vi "002_NBT Testplatform V3.1.vi"(11 "Queue Ref In":T1={"UI"=refnum, "Message"=refnum, "Data"=refnum, "Caller"=refnum, "Name"="000 Common", "Data Path"=path "", "Class Path"=path "", "SubPanel"=refnum, "Project Name"="", "MNT"="", "Title"="", "Data Source"=refnum, "Queue List"={}, "VI"=refnum, "UE"=refnum}) -> ()   [LabVIEW 2020]
doc: "000001"
uses:
  Alin/QMH/000 Module Data Type.ctl
  Alin/QMH/Queue Message.ctl
  <vilib>/Utility/file.llb/Read Delimited Spreadsheet (string).vi
  <vilib>/Utility/file.llb/Write Delimited Spreadsheet (string).vi
  <vilib>/Utility/cursorutil.llb/Set Cursor (Icon Pict).vi
  <vilib>/Utility/config.llb/Read Key (String).vi
  <vilib>/Utility/config.llb/NI_LVConfig.lvlib
panel:
  in  "Data Source Manage":bool
  out "Logo":picture
  out "Title":string="AlinFramwork Test"
  out "Warning":bool
  in  "User":string="你好！管理员 Debug"
  out "Log":string
  in  "Warning Record":string
  out "字符串":string
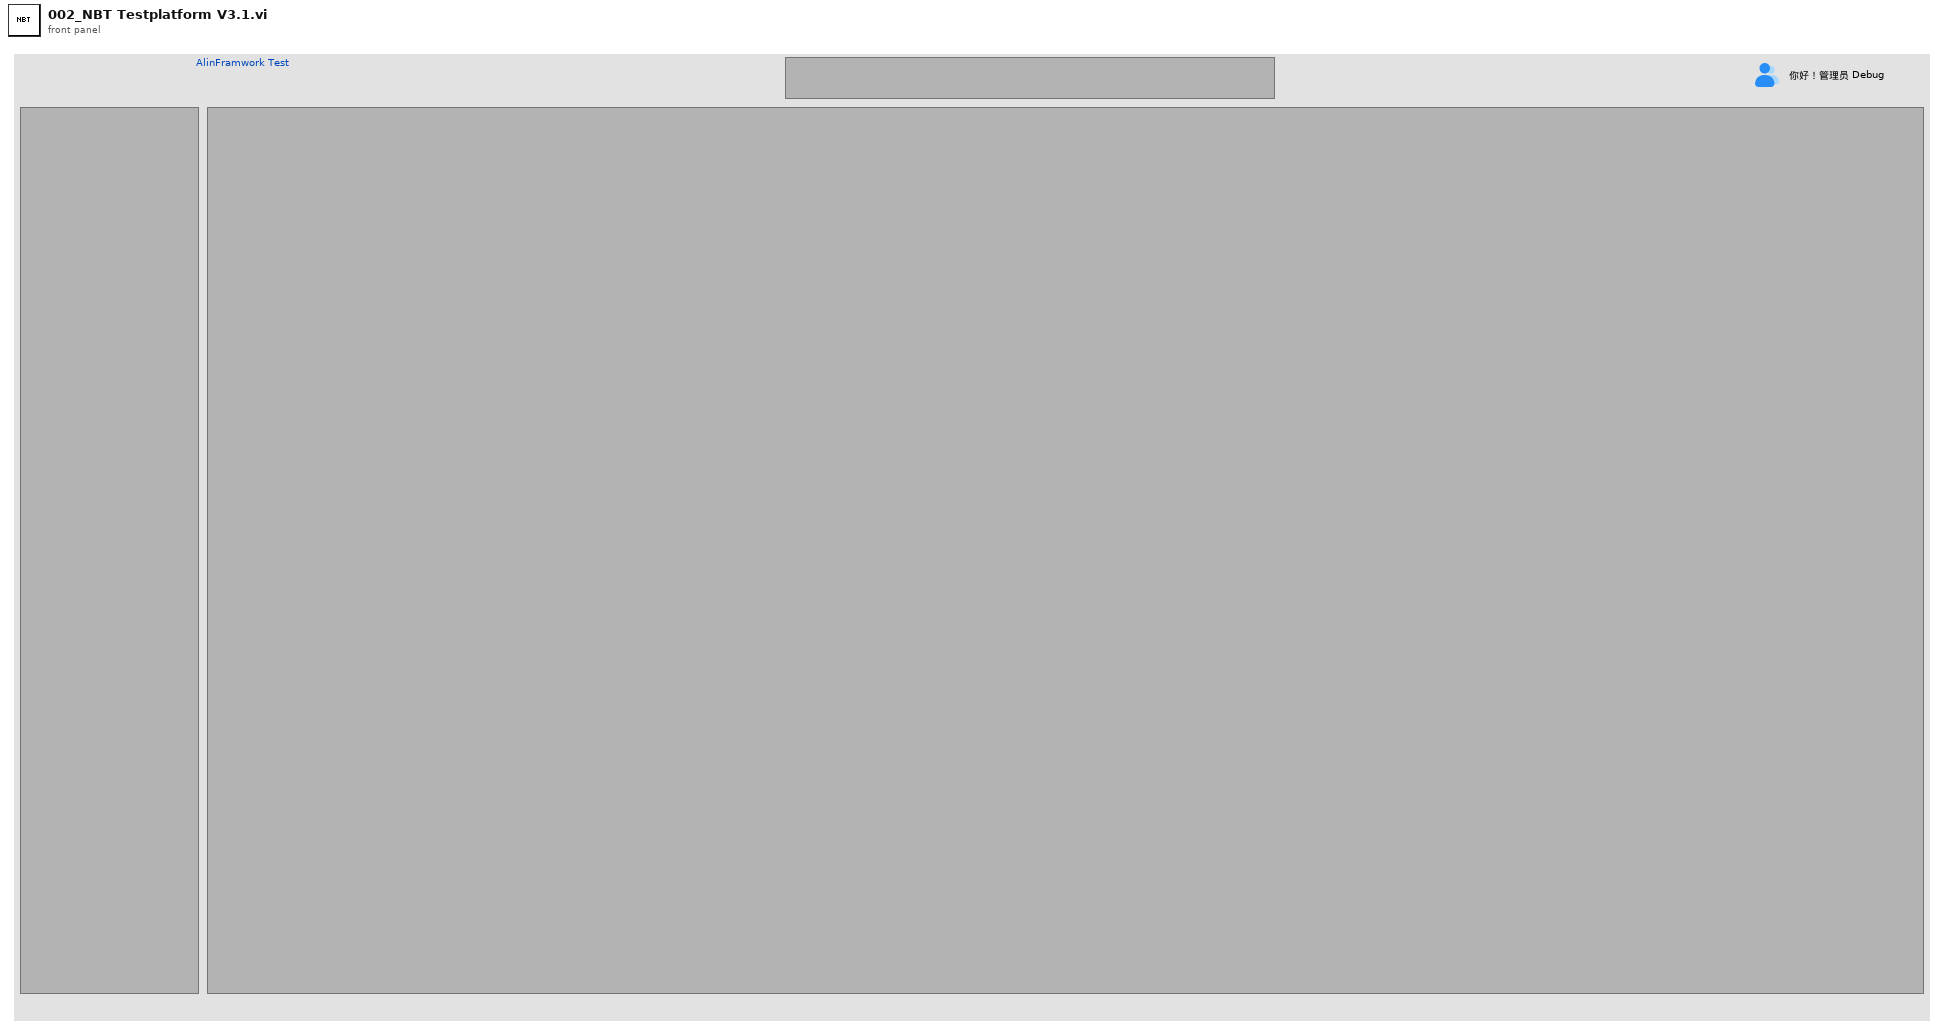
[diagram p1: front panel]
types:
  T1 = typedef "000 Module Data Type.ctl" = cluster{"UI":refnum<queue>, "Message":refnum<queue>, "Data":refnum<queue>, "Caller":refnum<queue>, "Name":string, "Data Path":path, "Class Path":path, "SubPanel":refnum<vi>, "Project Name":string, "MNT":string, "Title":string, "Data Source":refnum<queue>, "Queue List":map{string, refnum<queue>}, "VI":refnum<vi>, "UE":refnum<user-event>}
  T2 = cluster{"Interval":cluster{"min":i32, "max":i32}, "Color":cluster{"off":u32, "on":u32}, "Panel":cluster{"Panel01":bool, "Panel02":bool, "Panel03":bool, "Panel04":bool, "Panel05":bool, "Panel06":bool, "Panel07":bool}, "SubPanel":cluster{"Panel01":refnum<vi>, "Panel02":refnum<vi>, "Panel03":refnum<vi>, "Panel04":refnum<vi>, "Panel05":refnum<vi>, "Panel06":refnum<vi>, "Panel07":refnum<vi>}, "Queue Ref ":T1, "Panel Name":string[], "Write":map{string, string}, "Warning":refnum<vi>, "Info":cluster{"Title":string, "Names":string[], "Logo":string}, "Panel Config":bool, "Spliter":refnum<vi>, "Log Name":string, "Last":i32}
  T3 = typedef "NI_LVConfig.lvlib/Config Data RefNum.ctl" = refnum<k1>
  T4 = typedef "imagedata.ctl" = cluster{"image type":i32, "image depth":i32, "image":u8[], "mask":u8[], "colors":u32[], "Rectangle":cluster{"left":i16, "top":i16, "right":i16, "bottom":i16}}
  T5 = cluster{"Panel01":refnum<vi>, "Panel02":refnum<vi>, "Panel03":refnum<vi>, "Panel04":refnum<vi>, "Panel05":refnum<vi>, "Panel06":refnum<vi>, "Panel07":refnum<vi>}
  T6 = enum32{"invalid app kind", "Development System", "Run Time System", "Student Edition", "Embedded LabVIEW", "Evaluation", "Custom"}
  T7 = typedef "eventvkey.ctl" = enum16{"ASCII", "Enter", "Return", "Shift", "Ctrl", "Alt", "Cmd", "Opt", "Caps", "NumLock", "Clear", "Break", "Up", "Down", "Left", "Right", "Insert", "Delete", "Home", "End", "PageUp", "PageDown", "Escape", "Help", "Pause", "ScrollLock", "F1", "F2", "F3", "F4", "F5", "F6", "F7", "F8", "F9", "F10", "F11", "F12", "F13", "F14", "F15", "F16", "F17", "F18", "F19", "F20", "F21", "F22", "F23", "F24", "Play", "VolumeUp", "VolumeDown", "Mute", "Two Byte Char"}
  T8 = cluster{"Shift":bool, "Ctrl":bool, "Alt":bool, "Cmd":bool, "Opt":bool}
  T9 = cluster{"Queue Ref":T1, "Queue List":map{string, refnum<queue>}, "Panel Adjust":string, "Panel Name":string[], "Panel Info":map{string, cluster{"Lable":string, "Name":string, "Panel":string, "Use":string}}, "SubPanel":refnum<vi>}
  T10 = map{string, cluster{"Lable":string, "Name":string, "Panel":string, "Use":string}}
  T11 = cluster{"Lable":string, "Name":string, "Panel":string, "Use":string}
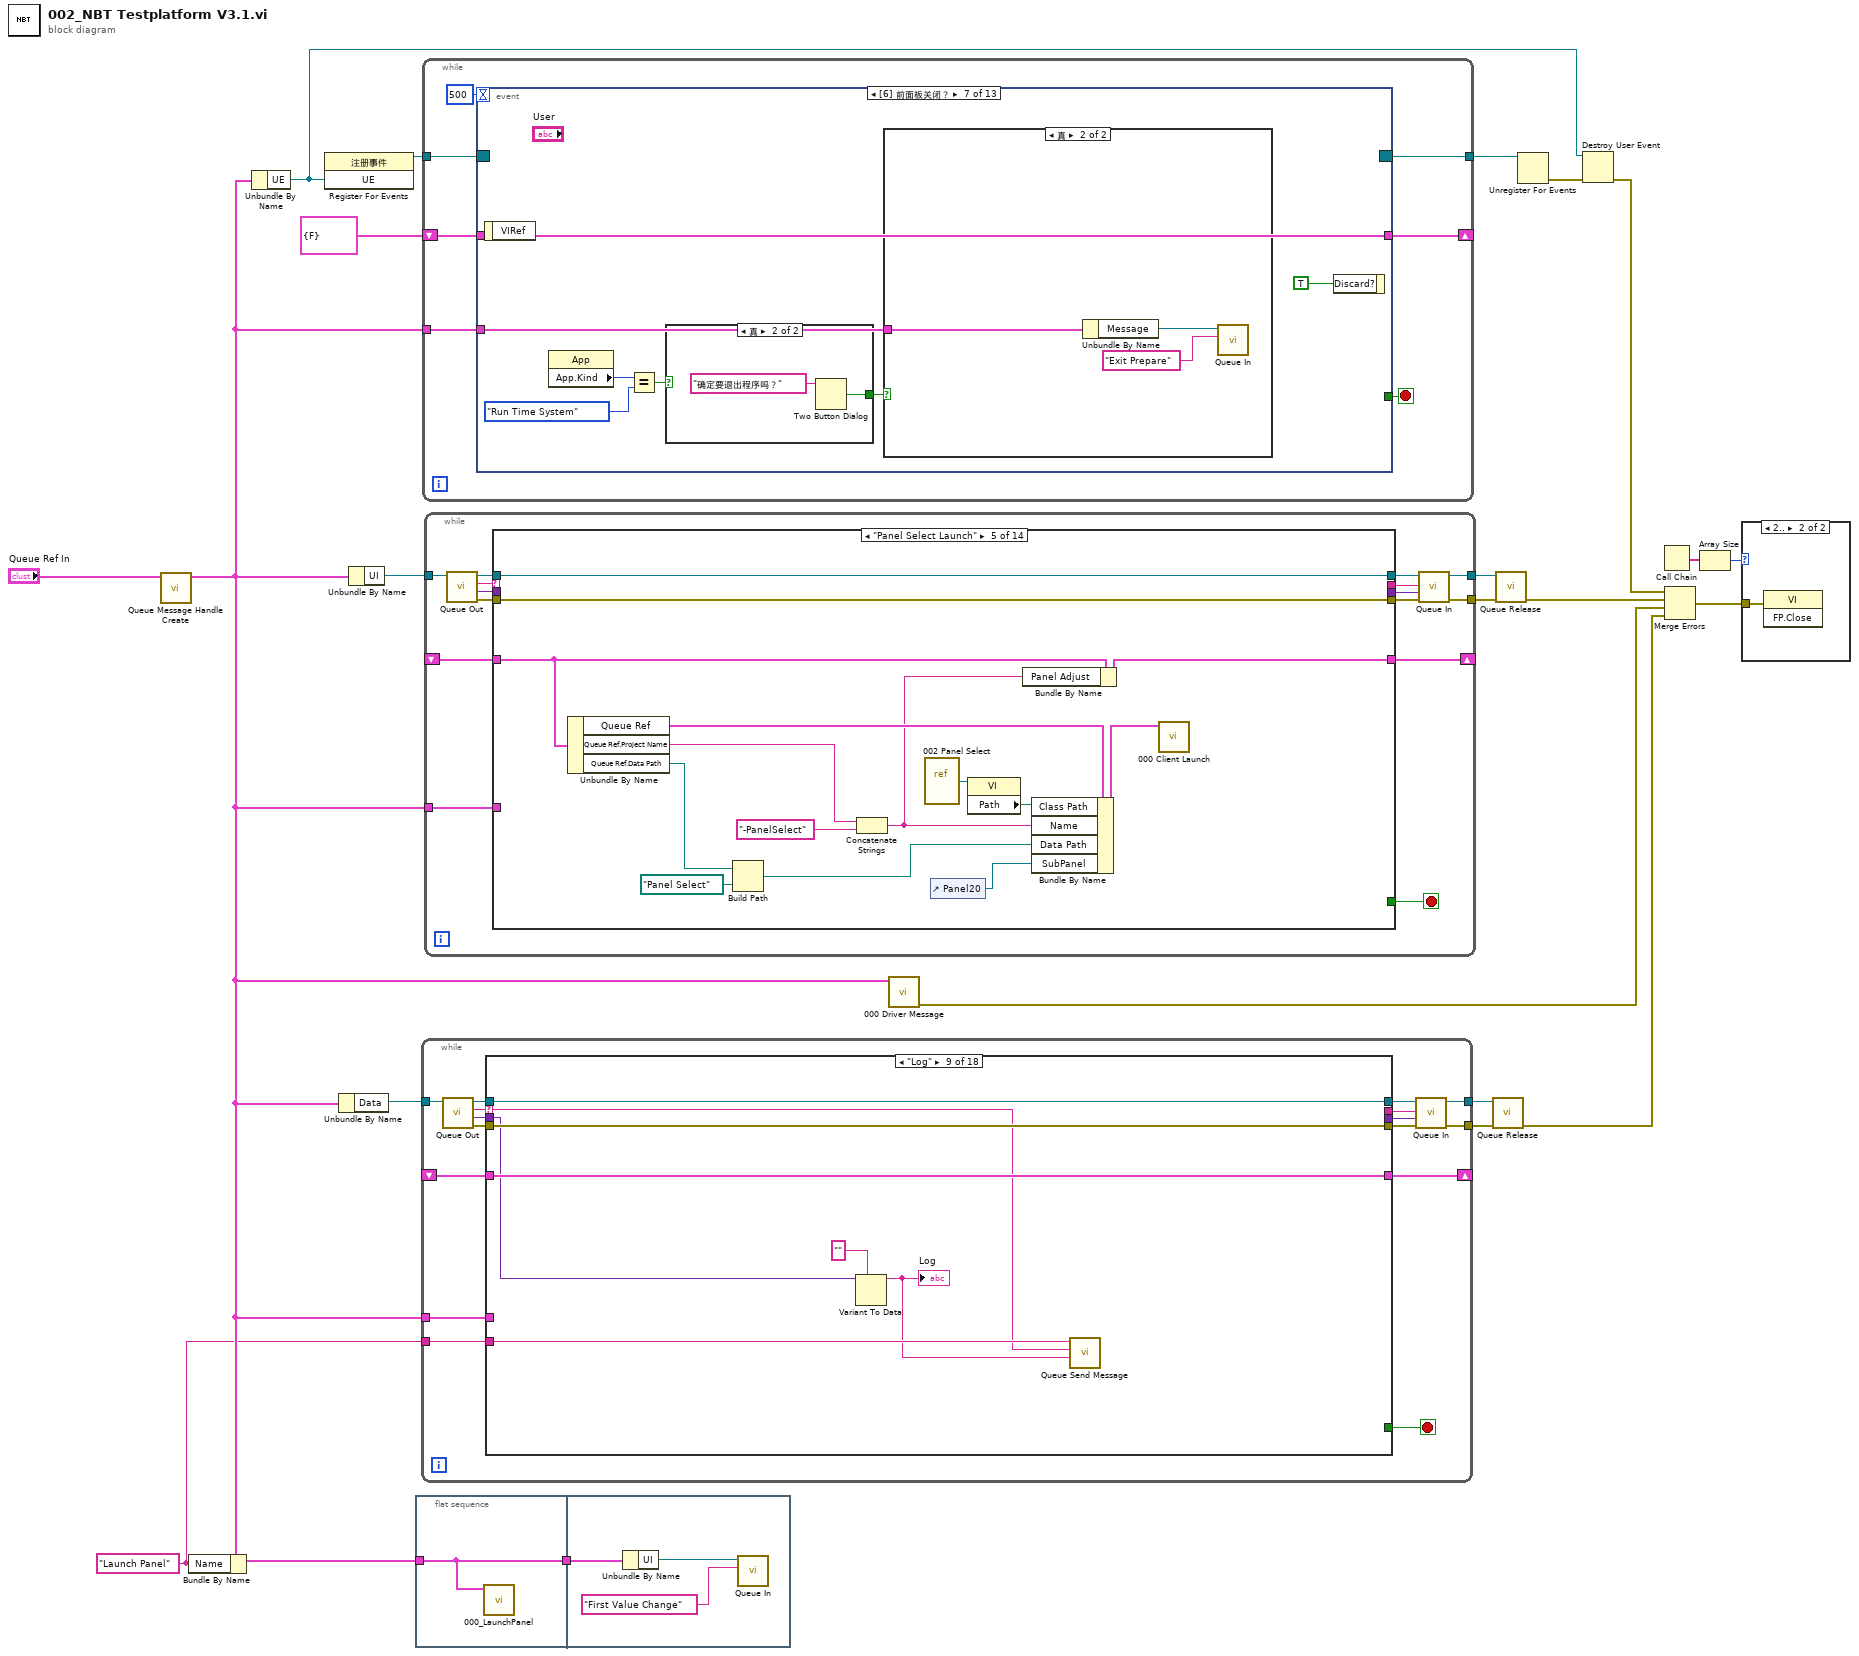
[diagram p0: block diagram]
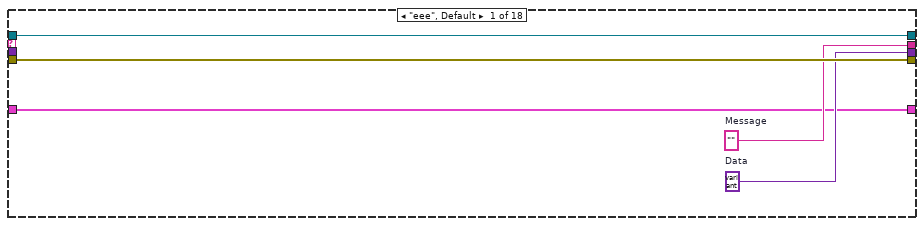
[diagram p2: hidden frame]
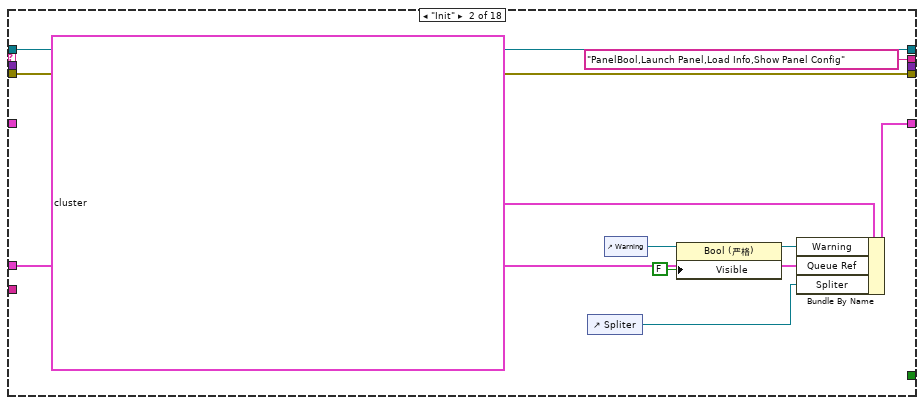
[diagram p3: hidden frame]
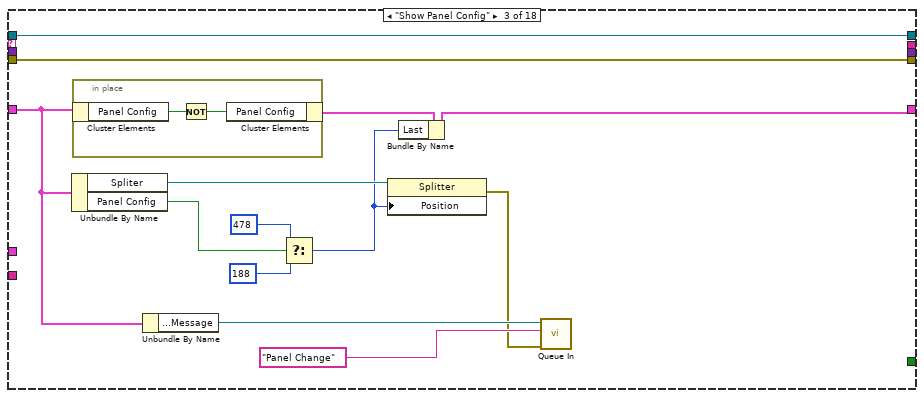
[diagram p4: hidden frame]
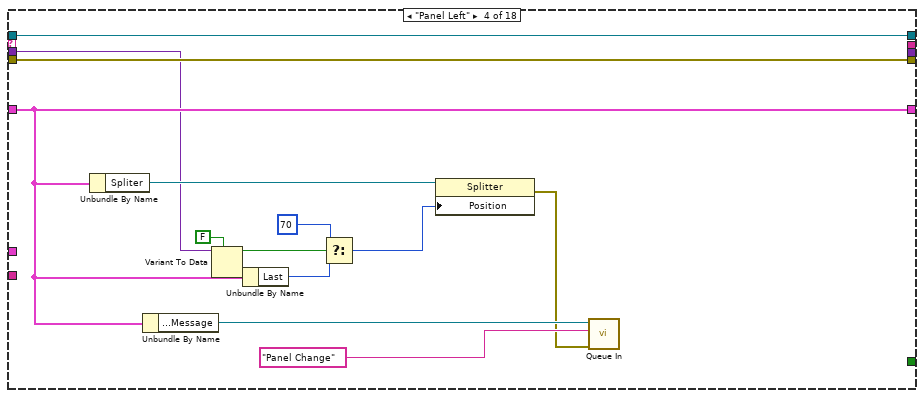
[diagram p5: hidden frame]
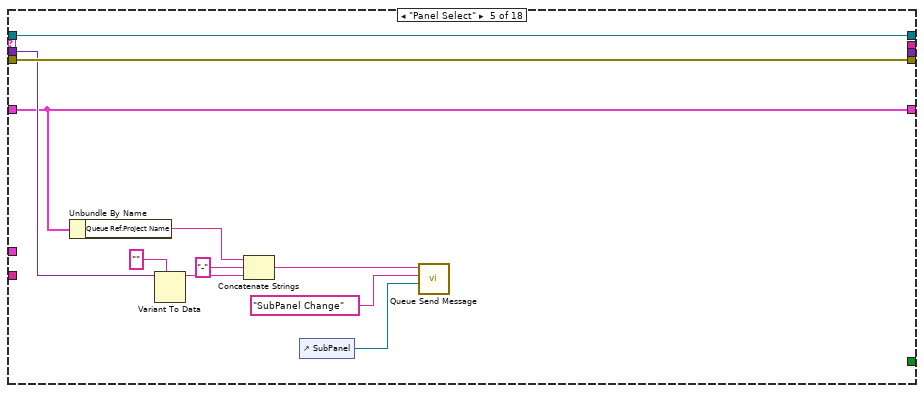
[diagram p6: hidden frame]
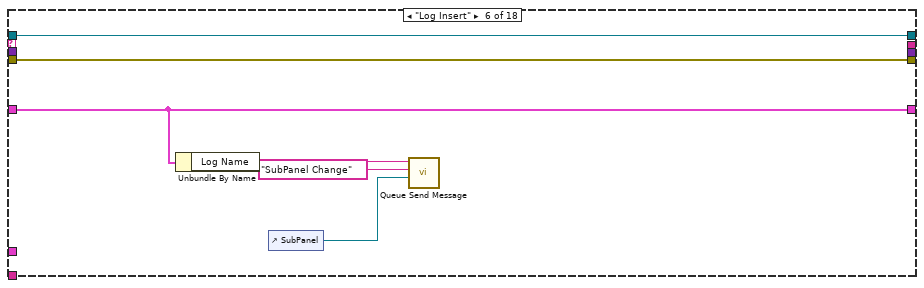
[diagram p7: hidden frame]
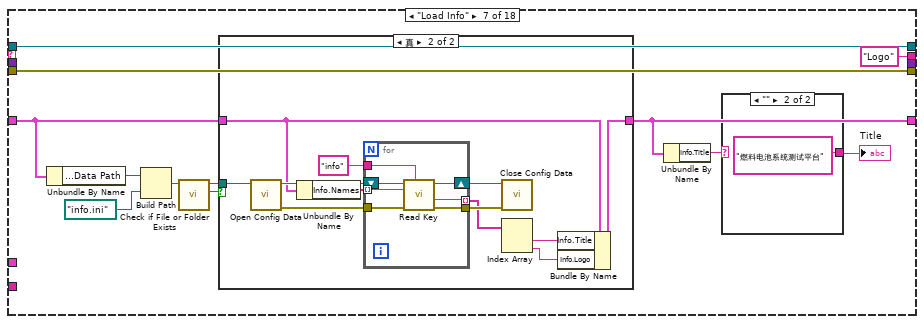
[diagram p8: hidden frame]
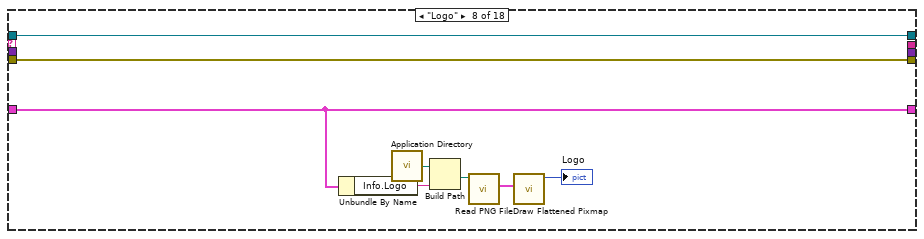
[diagram p11: hidden frame]
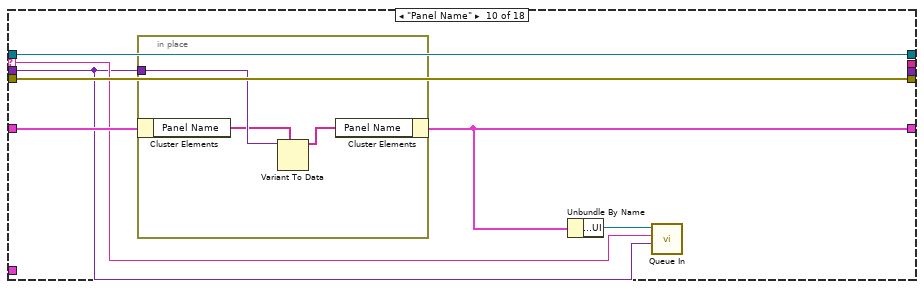
[diagram p12: hidden frame]
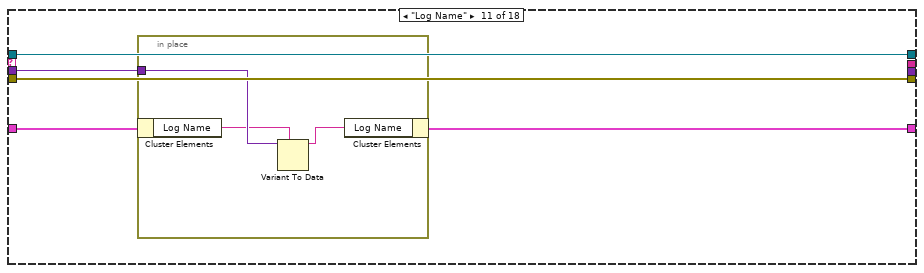
[diagram p13: hidden frame]
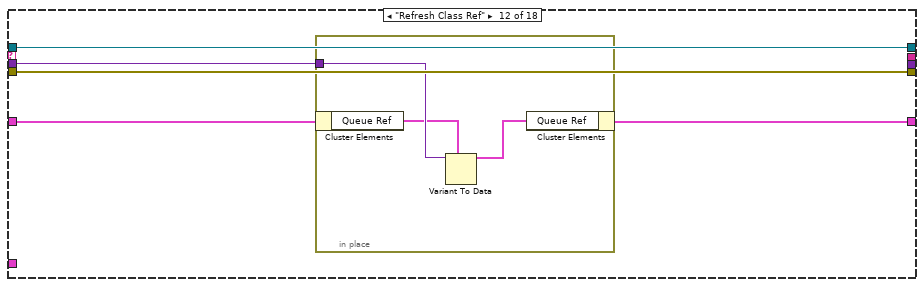
[diagram p14: hidden frame]
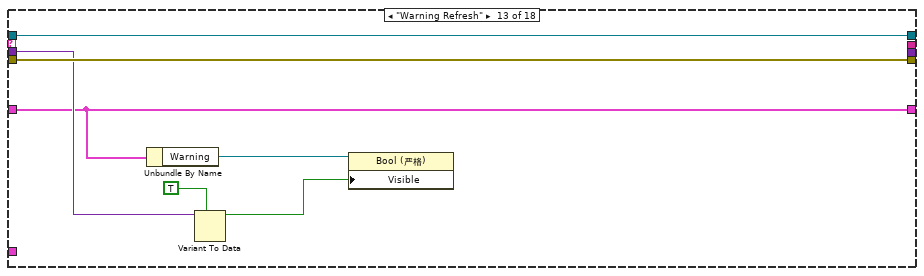
[diagram p15: hidden frame]
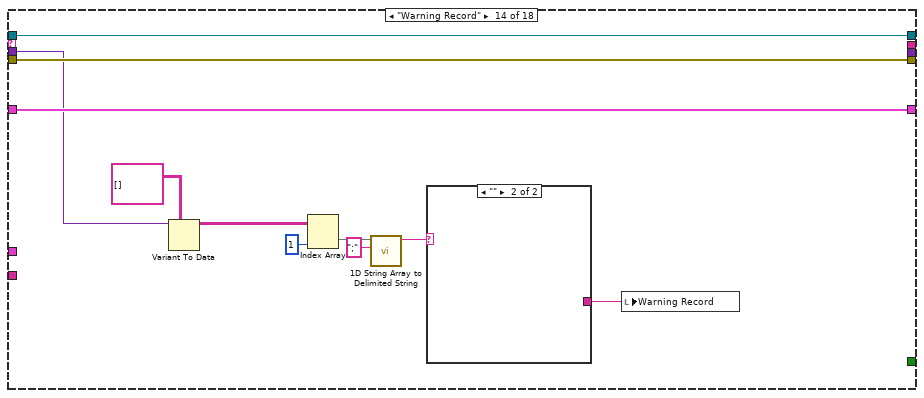
[diagram p16: hidden frame]
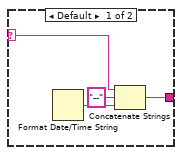
[diagram p17: hidden frame]
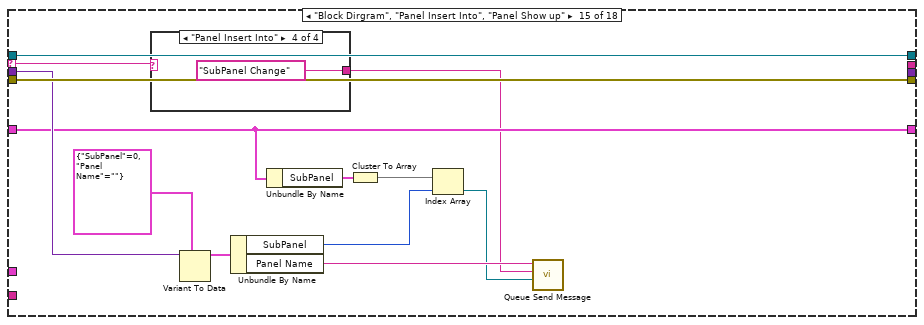
[diagram p18: hidden frame]
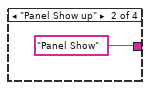
[diagram p20: hidden frame]
diagram:
  w2 = "Launch Panel" ("Name")
  n1 = call "Queue Message Handle Create.vi"("Queue Ref In"="Queue Ref In") -> ("Queue Ref Out"=w4:T1)  [unwired: 9 in, 1 out]
  n2 = Bundle By Name(cluster=w4, "Name"=w2) -> (w3:T1)
  n3 = Unbundle By Name(w4) -> ("UE"=w6:refnum<user-event>)
  n4 = register-events(w6) -> (reference out=w7:refnum<event-registration>)  [unwired: 2 in, 1 out]
  n5 = Unbundle By Name(w4) -> ("Data"=w20:refnum<queue>)
  n6 = Unbundle By Name(w4) -> ("UI"=w12:refnum<queue>)
  n7 = flat-sequence {
    tunnel: w3 -> [w24]
    tunnel: [w24] -> w1
    tunnel: w1 -> [w27]
    frame #0 {
      n8 = call "000_LaunchPanel.vi"("Queue Ref In"=w24) -> ()  [unwired: 11 in]
    }
    frame #1 {
      n9 = Unbundle By Name(w27) -> ("UI"=w26:refnum<queue>)
      n10 = call "Queue In.vi"("Message"="First Value Change", "Queue In"=w26) -> ()  [unwired: 8 in, 2 out]
    }
  }
  n11 = while {
    tunnel: w20 -> [w39]
    tunnel: [w36] -> w18
    tunnel: [w35] -> w19
    shift-right: [w31] -> _
    shift-left: _ -> [w30]
    tunnel: w4 -> [w29]
    tunnel: w2 -> [w28]
    stop <- w43 stop-if-true
    n12 = call "Queue Out.vi"("Queue In"=w39) -> ("error out"=w42:errorcluster, "Data"=w40:variant, "Message"=w41:string, "Queue Out"=w38:refnum<queue>)  [unwired: 6 in, 1 out]
    n13 = case shown="\"Log\"" w41 {
      selector: w41 -> [_ _ _ _ _ _ _ _ w146 w155 _ _ _ _ w203 _ _ _]
      tunnel: w38 -> [w48 w58 w71 w86 w97 w103 w115 w145 w153 w160 w168 w176 w186 w197 w214 w222 w227 w231]
      tunnel: w42 -> [w47 w57 w70 w85 w96 w102 w114 w144 w152 w159 w167 w175 w185 w196 w213 w221 w225 w232]
      tunnel: [w48 w58 w71 w86 w97 w103 w115 w145 w153 w160 w168 w176 w186 w197 w214 w222 w226 w231] -> w37
      tunnel: [w47 w57 w70 w85 w96 w102 w114 w144 w152 w159 w167 w175 w185 w196 w213 w221 w224 w232] -> w34
      tunnel: [w46 "PanelBool,Launch Panel,Load Info,Show Panel Config" ("Message") _ _ _ _ "Logo" ("Message") _ _ _ _ _ _ _ _ _ "Quit" _] -> w33
      tunnel: [_ _ _ _ _ _ _ _ _ _ _ _ _ _ _ _ _ TRUE] -> w43
      tunnel: [w45 _ _ _ _ _ _ _ _ _ _ _ _ _ _ _ _ _] -> w32
      tunnel: w40 -> [_ _ _ w76 w95 _ _ _ w150 w154 w164 w172 w184 w194 w212 _ _ _]
      tunnel: [w44 w54 w60 w78 w93 w101 w107 w139 w151 w157 w165 w173 w182 w195 w209 w220 w223 w229] -> w31
      tunnel: w30 -> [w44 _ w64 w78 w93 w101 w108 w139 w151 w158 w166 w174 w182 w195 w209 w220 w223 w229]
      tunnel: w29 -> [_ w50 _ _ _ _ _ _ _ _ _ _ _ _ _ _ _ _]
      tunnel: w28 -> [_ _ _ _ _ _ _ _ w148 _ _ _ _ _ _ _ _ _]
      frame "eee", Default {
        w45 = variant  # Data
        w46 = ""  # Message
      }
      frame "Init" {
        n14 = control-ref of="Spliter"() -> (w49:refnum<vi>)
        n15 = control-ref of="Warning"() -> (w53:refnum<vi>)
        n16 = property class="Bool (严格)"(reference=w53, "Visible"=FALSE ("可见")) -> (reference out=w52:refnum<vi>)  [unwired: 1 in, 1 out]
        n17 = Bundle By Name(cluster=T2 {"Interval"={"min"=3, "max"=300}, "Color"={"off"=16777225, "on"=16777238}, "Panel"={"Panel01"=FALSE, "Panel02"=FALSE, "Panel03"=FALSE, "Panel04"=FALSE, "Panel05"=FALSE, "Panel06"=FALSE, "Panel07"=FALSE}, "SubPanel"={"Panel01"=refnum, "Panel02"=refnum, "Panel03"=refnum, "Panel04"=refnum, "Panel05"=refnum, "Panel06"=refnum, "Panel07"=refnum}, "Queue Ref "={"UI"=refnum, "Message"=refnum, "Data"=refnum, "Caller"=refnum, "Name"="000 Common", "Data Path"=path "", "Class Path"=path "", "SubPanel"=refnum, "Project Name"="", "MNT"="", "Title"="", "Data Source"=refnum, "Queue List"={}, "VI"=refnum, "UE"=refnum}, "Panel Name"=[], "Write"={}, "Warning"=refnum, "Info"={"Title"="", "Names"=["Title", "Logo"], "Logo"=""}, "Panel Config"=FALSE, "Spliter"=refnum, "Log Name"="", "Last"=188}, "Warning"=w52, "Queue Ref"=w50, "Spliter"=w49) -> (w54:T2)
      }
      frame "Show Panel Config" {
        n18 = Unbundle By Name(w64) -> ("Spliter"=w69:refnum<vi>, "Panel Config"=w68:bool)
        n19 = in-place {
          n20 = in-place-cluster #1(w64) -> ("Panel Config"=w73:bool)
          n21 = Not(x=w73) -> (.not. x?=w72:bool)
          n22 = in-place-cluster #1("Panel Config"=w72) -> (w65:T2)
        }
        n23 = Unbundle By Name(w64) -> ("Queue Ref.Message"=w63:refnum<queue>)
        n24 = Select(t=478 ("分隔栏位置"), s=w68, f=188 ("分隔栏位置")) -> (s? t:f=w59:i32)
        n25 = property class="Splitter"(reference=w69, "Position"=w59) -> (error out=w61:errorcluster)  [unwired: 1 in, 1 out]
        n26 = Bundle By Name(cluster=w65, "Last"=w59) -> (w60:T2)
        n27 = call "Queue In.vi"("error in (no error)"=w61, "Message"="Panel Change", "Queue In"=w63) -> ()  [unwired: 7 in, 2 out]
      }
      frame "Panel Left" {
        n28 = Unbundle By Name(w78) -> ("Spliter"=w84:refnum<vi>)
        n29 = Unbundle By Name(w78) -> ("Queue Ref.Message"=w81:refnum<queue>)
        n30 = Variant To Data(type=FALSE, Variant=w76) -> (data=w74:bool)  [unwired: 1 in, 1 out]
        n31 = Unbundle By Name(w78) -> ("Last"=w77:i32)
        n32 = Select(t=70 ("分隔栏位置"), s=w74, f=w77) -> (s? t:f=w82:i32)
        n33 = property class="Splitter"(reference=w84, "Position"=w82) -> (error out=w79:errorcluster)  [unwired: 1 in, 1 out]
        n34 = call "Queue In.vi"("error in (no error)"=w79, "Message"="Panel Change", "Queue In"=w81) -> ()  [unwired: 7 in, 2 out]
      }
      frame "Panel Select" {
        n35 = Unbundle By Name(w93) -> ("Queue Ref.Project Name"=w92:string)
        n36 = Variant To Data(type="" ("元素"), Variant=w95) -> (data=w90:string)  [unwired: 1 in, 1 out]
        n37 = Concatenate Strings(w92, "-" ("字符串"), w90) -> (w89:string)
        n38 = control-ref of="SubPanel"() -> (w87:refnum<vi>)
        n39 = call "Queue Send Message.vi"("Data"=w87, "Message"="SubPanel Change", "Queue Name"=w89) -> ()  [unwired: 6 in, 3 out]
      }
      frame "Log Insert" {
        n40 = Unbundle By Name(w101) -> ("Log Name"=w100:string)
        n41 = control-ref of="SubPanel"() -> (w99:refnum<vi>)
        n42 = call "Queue Send Message.vi"("Data"=w99, "Message"="SubPanel Change", "Queue Name"=w100) -> ()  [unwired: 6 in, 3 out]
      }
      frame "Load Info" {
        n43 = Unbundle By Name(w108) -> ("Queue Ref.Data Path"=w113:path)
        n44 = Build Path(base path=w113, name or relative path=path "info.ini" ("名称或相对路径")) -> (appended path=w111:path)
        n45 = call <vilib>:"Check if File or Folder Exists.vi"("path"=w111) -> ("file or folder exists?"=w109:bool, "dup path"=w110:path)  [unwired: 8 in, 1 out]
        n46 = case shown="真" w109 {
          tunnel: w110 -> [_ w126]
          tunnel: w108 -> [w118 w125]
          tunnel: [w118 w122] -> w107
          frame False {
          }
          frame True {
            n47 = call <vilib>:"Open Config Data.vi"("configuration file path"=w126) -> ("error out"=w129:errorcluster, "refnum"=w130:T3)  [unwired: 8 in, 1 out]
            n48 = Unbundle By Name(w125) -> ("Info.Names"=w124:string[])
            n49 = for {
              tunnel: w129 -> [w136]
              tunnel: [w134] -> w127
              shift-right: [w135] -> w128
              shift-left: w130 -> [w137]
              tunnel: w124 -> [w133] mode=indexing
              tunnel: [w132] -> w123 mode=indexing
              tunnel: "info" ("section") -> [w131]
              n50 = call-poly <vilib>:"Read Key.vi"("section"=w131, "error in (no error)"=w136, "key"=w133, "refnum"=w137) -> ("error out"=w134:errorcluster, "value"=w132:string, "refnum out"=w135:T3)  [unwired: 4 in, 1 out]
            }
            n51 = call <vilib>:"Close Config Data.vi"("error in (no error)"=w127, "refnum"=w128) -> ()  [unwired: 8 in, 2 out]
            n52 = Index Array(array=w123) -> (element #1=w121:string, element #2=w119:string)  [unwired: 2 in]
            n53 = Bundle By Name(cluster=w125, "Info.Title"=w121, "Info.Logo"=w119) -> (w122:T2)
          }
        }
        n54 = Unbundle By Name(w107) -> ("Info.Title"=w106:string)
        n55 = case shown="\"\"" w106 {
          selector: w106 -> [w116 _]
          tunnel: [w116 "燃料电池系统测试平台"] -> w105
          frame Default {
          }
          frame "" {
          }
        }
        "Title" <- w105
      }
      frame "Logo" {
        n56 = Unbundle By Name(w139) -> ("Info.Logo"=w138:string)
        n57 = call <vilib>:"Application Directory.vi"() -> ("Application Directory"=w140:path)
        n58 = Build Path(base path=w140, name or relative path=w138) -> (appended path=w141:path)
        n59 = call <vilib>:"Read PNG File.vi"("path to PNG file"=w141) -> ("image data"=w142:T4)  [unwired: 8 in, 2 out]
        n60 = call <vilib>:"Draw Flattened Pixmap.vi"("image data"=w142) -> ("new picture"=→"Logo":picture)  [unwired: 8 in]
      }
      frame "Log" {
        n61 = Variant To Data(type="", Variant=w150) -> (data=w147:string)  [unwired: 1 in, 1 out]
        "Log" <- w147
        n62 = call "Queue Send Message.vi"("Data"=w147, "Message"=w146, "Queue Name"=w148) -> ()  [unwired: 6 in, 3 out]
      }
      frame "Panel Name" {
        n63 = in-place {
          in-place-border: w154 -> [w163]
          n64 = in-place-cluster #2(w158) -> ("Panel Name"=w162:string[])
          n65 = Variant To Data(type=w162, Variant=w163) -> (data=w161:string[])  [unwired: 1 in, 1 out]
          n66 = in-place-cluster #2("Panel Name"=w161) -> (w157:T2)
        }
        n67 = Unbundle By Name(w157) -> ("Queue Ref.UI"=w156:refnum<queue>)
        n68 = call "Queue In.vi"("Data"=w154, "Message"=w155, "Queue In"=w156) -> ()  [unwired: 7 in, 2 out]
      }
      frame "Log Name" {
        n69 = in-place {
          in-place-border: w164 -> [w171]
          n70 = in-place-cluster #3(w166) -> ("Log Name"=w170:string)
          n71 = Variant To Data(type=w170, Variant=w171) -> (data=w169:string)  [unwired: 1 in, 1 out]
          n72 = in-place-cluster #3("Log Name"=w169) -> (w165:T2)
        }
      }
      frame "Refresh Class Ref" {
        n73 = in-place {
          in-place-border: w172 -> [w179]
          n74 = in-place-cluster #4(w174) -> ("Queue Ref"=w178:T1)
          n75 = Variant To Data(type=w178, Variant=w179) -> (data=w177:T1)  [unwired: 1 in, 1 out]
          n76 = in-place-cluster #4("Queue Ref"=w177) -> (w173:T2)
        }
      }
      frame "Warning Refresh" {
        n77 = Unbundle By Name(w182) -> ("Warning"=w181:refnum<vi>)
        n78 = Variant To Data(type=TRUE, Variant=w184) -> (data=w180:bool)  [unwired: 1 in, 1 out]
        n79 = property class="Bool (严格)"(reference=w181, "Visible"=w180) -> ()  [unwired: 1 in, 2 out]
      }
      frame "Warning Record" {
        n80 = Variant To Data(type=string[][] [], Variant=w194) -> (data=w192:string[][])  [unwired: 1 in, 1 out]
        n81 = Index Array(array=w192, index (col)=1 ("禁用的索引 (列)")) -> (element=w190:string[])  [unwired: 1 in]
        n82 = call <vilib>:"1D String Array to Delimited String.vi"("delimiter"=";", "string array"=w190) -> ("delimited string"=w188:string)  [unwired: 9 in]
        n83 = case shown="\"\"" w188 {
          selector: w188 -> [w201 _]
          tunnel: [w198 _] -> w187
          frame Default {
            n84 = Format Date/Time String() -> (date/time string=w200:string)  [unwired: 3 in]
            n85 = Concatenate Strings(w201, "--" ("字符串"), w200) -> (w198:string)
          }
          frame "" {
          }
        }
        n86 = local write "Warning Record"(w187) -> ()
      }
      frame "Block Dirgram", "Panel Insert Into", "Panel Show up" {
        n87 = case shown="\"Panel Insert Into\"" w203 {
          tunnel: [_ "Panel Show" ("Message") "Show Block Dirgram" ("Message") "SubPanel Change" ("Message")] -> w202
          frame "假", Default {
          }
          frame "Panel Show up" {
          }
          frame "Block Dirgram" {
          }
          frame "Panel Insert Into" {
          }
        }
        n88 = Variant To Data(type=cluster{"SubPanel":i32, "Panel Name":string} {"SubPanel"=0, "Panel Name"=""} ("簇"), Variant=w212) -> (data=w210:cluster{"SubPanel":i32, "Panel Name":string})  [unwired: 1 in, 1 out]
        n89 = Unbundle By Name(w210) -> ("SubPanel"=w206:i32, "Panel Name"=w205:string)
        n90 = Unbundle By Name(w209) -> ("SubPanel"=w208:T5)
        n91 = Cluster To Array(cluster=w208) -> (array=w207:refnum<vi>[])
        n92 = Index Array(array=w207, index=w206) -> (element=w204:refnum<vi>)
        n93 = call "Queue Send Message.vi"("Data"=w204, "Message"=w202, "Queue Name"=w205) -> ()  [unwired: 6 in, 3 out]
      }
      frame "Caller Exit" {
        n94 = Unbundle By Name(w220) -> ("Queue Ref.Caller"=w219:refnum<queue>)
        n95 = call "Queue In.vi"("Message"="Exit Prepare", "Queue In"=w219) -> ()  [unwired: 8 in, 2 out]
      }
      frame "Exit" {
        n96 = call "Queue Clear.vi"("error in (no error)"=w225, "Queue In"=w227) -> ("error out"=w224:errorcluster, "Queue Out"=w226:refnum<queue>)  [unwired: 8 in]
      }
      frame "Quit" {
      }
    }
    n97 = call "Queue In.vi"("error in (no error)"=w34, "Data"=w32, "Message"=w33, "Queue In"=w37) -> ("error out"=w35:errorcluster, "Queue Out"=w36:refnum<queue>)  [unwired: 6 in]
  }
  n98 = while {
    tunnel: w7 -> [w239]
    tunnel: [w237] -> w8
    tunnel: w4 -> [w236]
    shift-right: [w233] -> _
    shift-left: cluster{"Warning":bool} {"Warning"=FALSE} -> [w234]
    stop <- w238 stop-if-true
    n99 = event shown="[6] 前面板关闭？" {
      selector: w239 -> [_ _ _ _ _ _ _ _ _ _ _ _ _]
      dyn-events: [_ _ _ _ _ _ _ _ _ _ _ _ _] -> w237
      timeout: 500 -> [_ _ _ _ _ _ _ _ _ _ _ _ _]
      tunnel: [_ _ _ _ _ w261 _ _ _ _ _ _ _] -> w238
      tunnel: w236 -> [_ _ _ w250 w259 _ w269 w277 w284 w293 _ _ w304]
      tunnel: w234 -> [w242 w247 w249 w255 w256 w260 w264 w278 w283 w289 w300 w302 w305]
      tunnel: [w241 w247 w249 w255 w256 w260 w264 w278 w283 w289 w300 w302 w305] -> w233
      event Timeout {
        n100 = event-data() -> ()  [unwired: 1 in, 1 out]
        n101 = Format Date/Time String() -> (date/time string=→"字符串":string)  [unwired: 3 in]
        n102 = in-place {
          in-place-border: [w244] -> w240
          n103 = in-place-cluster #5(w242) -> ("Warning"=w245:bool)
          n104 = Not(x=w245) -> (.not. x?=w244:bool)
          n105 = in-place-cluster #5("Warning"=w244) -> (w241:cluster{"Warning":bool})
        }
        "Warning" <- w240
      }
      event "Warning Record": Mouse Enter {
        n106 = event-data() -> ()  [unwired: 1 in, 1 out]
        n107 = call-poly <vilib>:"Set Cursor.vi"("icon"=u16 6) -> ()  [unwired: 9 in, 2 out]
      }
      event "Warning Record": Mouse Leave {
        n108 = event-data() -> ()  [unwired: 1 in, 1 out]
        n109 = call-poly <vilib>:"Set Cursor.vi"("icon"=u16 0) -> ()  [unwired: 9 in, 2 out]
      }
      event Key Down {
        n110 = event-data() -> ("Char"=w254:i16, "VKey"=w253:T7, "Mods"=w252:cluster{"Num Pad":bool, "Menu Key":bool}, "PlatMods"=w251:T8)  [unwired: 1 in]
        n111 = call "Queue Key Down.vi"("Queue Ref Out"=w250, "C"=w254, "Platform Key"=w251, "Group Key"=w252, "V Key"=w253) -> ()  [unwired: 6 in, 1 out]
      }
      event Panel Resize {
        n112 = event-data() -> ()  [unwired: 1 in, 1 out]
        n113 = Unbundle By Name(w259) -> ("Message"=w258:refnum<queue>)
        n114 = call "Queue In.vi"("Message"="Panel Change", "Queue In"=w258) -> ()  [unwired: 8 in, 2 out]
      }
      event User Event {
        n115 = event-data() -> ("Message"=w263:string)  [unwired: 1 in]
        n116 = Equal?(x=w263, y="Exit") -> (x = y?=w261:bool)
      }
      event Panel Close? {
        n117 = event-data() -> ()  [unwired: 1 in, 1 out]
        n118 = property class="App"() -> ("App.Kind"=w268:T6)  [unwired: 2 in, 2 out]
        n119 = Equal?(x=w268, y=T6."Run Time System") -> (x = y?=w267:bool)
        n120 = case shown="真" w267 {
          tunnel: [TRUE ("T button?") w275] -> w265
          frame False {
          }
          frame True {
            n121 = Two Button Dialog(message="确定要退出程序吗？" ("消息")) -> (T button?=w275:bool)  [unwired: 2 in]
          }
        }
        n122 = case shown="真" w265 {
          tunnel: w269 -> [_ w273]
          frame False {
          }
          frame True {
            n123 = Unbundle By Name(w273) -> ("Message"=w272:refnum<queue>)
            n124 = call "Queue In.vi"("Message"="Exit Prepare", "Queue In"=w272) -> ()  [unwired: 8 in, 2 out]
          }
        }
        n125 = event-data("Discard?"=TRUE ("放弃？")) -> ()  [unwired: 1 in, 1 out]
      }
      event "Warning": Mouse Down {
        n126 = event-data() -> ("Mods.Double Click"=w279:bool)  [unwired: 1 in, 1 out]
        n127 = case shown="真" w279 {
          tunnel: w277 -> [_ w282]
          frame False {
          }
          frame True {
            n128 = Unbundle By Name(w282) -> ("Data"=w281:refnum<queue>)
            n129 = call "Queue In.vi"("Message"="Log Insert", "Queue In"=w281) -> ()  [unwired: 8 in, 2 out]
          }
        }
      }
      event "Title": Mouse Down {
        n130 = event-data() -> ("Mods.Double Click"=w285:bool)  [unwired: 1 in]
        n131 = case shown="真" w285 {
          tunnel: w284 -> [_ w288]
          frame False {
          }
          frame True {
            n132 = Unbundle By Name(w288) -> ("UI"=w287:refnum<queue>)
            n133 = call "Queue In.vi"("Message"="FCTS DAQ", "Queue In"=w287) -> ()  [unwired: 8 in, 2 out]
          }
        }
      }
      event "Data Source Manage": Mouse Down {
        n134 = event-data() -> ("CtlRef"=w294:refnum<vi>, "Mods.Double Click"=w292:bool, "PlatMods.Ctrl"=w291:bool)  [unwired: 1 in, 2 out]
        n135 = And(x=w292, y=w291) -> (x .and. y?=w290:bool)
        n136 = case shown="真" w290 {
          tunnel: w294 -> [_ w298]
          tunnel: w293 -> [_ w297]
          frame False {
          }
          frame True {
            n137 = property class="Bool (严格)"(reference=w298) -> ("Label.Text"=w295:string)  [unwired: 1 in, 2 out]
            n138 = Unbundle By Name(w297) -> ("UI"=w296:refnum<queue>)
            n139 = call "Queue In.vi"("Message"=w295, "Queue In"=w296) -> ()  [unwired: 8 in, 2 out]
          }
        }
      }
      event "Title": Mouse Enter {
        n140 = event-data() -> ()  [unwired: 1 in, 1 out]
        n141 = call-poly <vilib>:"Set Cursor.vi"("icon"=u16 6) -> ()  [unwired: 9 in, 2 out]
      }
      event "Title": Mouse Leave {
        n142 = event-data() -> ()  [unwired: 1 in, 3 out]
        n143 = call-poly <vilib>:"Set Cursor.vi"("icon"=u16 0) -> ()  [unwired: 9 in, 2 out]
      }
      event "Warning Record": Mouse Down {
        n144 = event-data() -> ("Mods.Double Click"=w303:bool)  [unwired: 1 in]
        n145 = case shown="真" w303 {
          tunnel: w304 -> [_ w308]
          frame False {
          }
          frame True {
            n146 = Unbundle By Name(w308) -> ("Data"=w307:refnum<queue>)
            n147 = call "Queue In.vi"("Message"="Log Insert", "Queue In"=w307) -> ()  [unwired: 8 in, 2 out]
          }
        }
      }
    }
  }
  n148 = while {
    tunnel: w12 -> [w319]
    tunnel: [w316] -> w10
    tunnel: [w315] -> w11
    shift-right: [w311] -> _
    shift-left: _ -> [w310]
    tunnel: w4 -> [w309]
    stop <- w323 stop-if-true
    n149 = call "Queue Out.vi"("Queue In"=w319) -> ("error out"=w322:errorcluster, "Data"=w320:variant, "Message"=w321:string, "Queue Out"=w318:refnum<queue>)  [unwired: 6 in, 1 out]
    n150 = case shown="\"Panel Select Launch\"" w321 {
      selector: w321 -> [_ _ _ _ _ w372 _ _ w400 _ _ _ w477 _]
      tunnel: w318 -> [w328 w335 w340 w356 w371 w376 w388 w394 w405 w418 w441 w468 w482 w488]
      tunnel: w322 -> [w327 w334 w339 w355 w370 w375 w387 w393 w404 w417 w440 w467 w480 w489]
      tunnel: [w328 w335 w340 w356 w371 w376 w388 w394 w405 w418 w441 w468 w481 w488] -> w317
      tunnel: [w327 w334 w339 w355 w370 w375 w387 w393 w404 w417 w440 w467 w479 w489] -> w314
      tunnel: [w326 "Launch Panel Adjust,Data Source Launch,Panel Info Load,Panel Select Launch" ("Message") _ _ _ _ _ _ "DeviceStatus" ("Message") w411 "Panel Refresh" ("Message") "Panel Info Load" ("Message") "Quit" _] -> w313
      tunnel: [_ _ _ _ _ _ _ _ _ _ _ _ _ TRUE] -> w323
      tunnel: [w325 _ _ _ _ _ _ _ _ _ _ _ _ _] -> w312
      tunnel: w320 -> [_ _ w337 _ _ _ _ _ w402 _ _ _ _ _]
      tunnel: [w324 w331 w336 w354 w358 w374 w386 w392 w401 w412 w434 w465 w475 w486] -> w311
      tunnel: w310 -> [w324 _ w338 w354 w369 w374 w386 w392 w403 w413 w438 w465 w475 w486]
      tunnel: w309 -> [_ w330 _ _ _ _ _ _ _ _ _ _ _ _]
      frame "eee", Default {
        w325 = variant  # Data
        w326 = ""  # Message
      }
      frame "Init" {
        n151 = control-ref of="SubPanel"() -> (w329:refnum<vi>)
        n152 = Bundle By Name(cluster=T9 {"Queue Ref"={"UI"=refnum, "Message"=refnum, "Data"=refnum, "Caller"=refnum, "Name"="000 Common", "Data Path"=path "", "Class Path"=path "", "SubPanel"=refnum, "Project Name"="", "MNT"="", "Title"="", "Data Source"=refnum, "Queue List"={}, "VI"=refnum, "UE"=refnum}, "Queue List"={}, "Panel Adjust"="", "Panel Name"=[], "Panel Info"={}, "SubPanel"=refnum}, "SubPanel"=w329, "Queue Ref"=w330) -> (w331:T9)
      }
      frame "Refresh Class Ref" {
        n153 = in-place {
          in-place-border: w337 -> [w343]
          n154 = in-place-cluster #6(w338) -> ("Queue Ref"=w342:T1)
          n155 = Variant To Data(type=w342, Variant=w343) -> (data=w341:T1)  [unwired: 1 in, 1 out]
          n156 = in-place-cluster #6("Queue Ref"=w341) -> (w336:T9)
        }
      }
      frame "Data Source Launch" {
        n157 = Unbundle By Name(w354) -> ("Queue Ref"=w353:T1, "Queue Ref.Project Name"=w349:string, "Queue Ref.Data Path"=w346:path)
        n158 = Build Path(base path=w346, name or relative path=path "Data Source" ("名称或相对路径")) -> (appended path=w344:path)
        n159 = Concatenate Strings(w349, "-DMS" ("Name")) -> (w347:string)
        n160 = vi-ref "002_Data Source Manage.vi"() -> (w352:refnum<vi>)
        n161 = property class="VI"(reference=w352) -> ("Path"=w350:path)  [unwired: 1 in, 2 out]
        n162 = Bundle By Name(cluster=w353, "Class Path"=w350, "Name"=w347, "Data Path"=w344) -> (w351:T1)
        n163 = call "000 Client Launch.vi"("Queue Ref"=w351) -> ()  [unwired: 10 in, 1 out]
      }
      frame "Panel Select Launch" {
        n164 = Unbundle By Name(w369) -> ("Queue Ref"=w368:T1, "Queue Ref.Project Name"=w364:string, "Queue Ref.Data Path"=w362:path)
        n165 = Build Path(base path=w362, name or relative path=path "Panel Select" ("名称或相对路径")) -> (appended path=w361:path)
        n166 = Concatenate Strings(w364, "-PanelSelect" ("Name")) -> (w357:string)
        n167 = vi-ref "002 Panel Select.vi"() -> (w367:refnum<vi>)
        n168 = control-ref of="Panel20"() -> (w359:refnum<vi>)
        n169 = property class="VI"(reference=w367) -> ("Path"=w365:path)  [unwired: 1 in, 2 out]
        n170 = Bundle By Name(cluster=w369, "Panel Adjust"=w357) -> (w358:T9)
        n171 = Bundle By Name(cluster=w368, "Class Path"=w365, "Name"=w357, "Data Path"=w361, "SubPanel"=w359) -> (w366:T1)
        n172 = call "000 Client Launch.vi"("Queue Ref"=w366) -> ()  [unwired: 10 in, 1 out]
      }
      frame "First Value Change" {
        n173 = Unbundle By Name(w374) -> ("Panel Adjust"=w373:string)
        n174 = call "Queue Send Message.vi"("Message"=w372, "Queue Name"=w373) -> ()  [unwired: 7 in, 3 out]
      }
      frame "Data Source Manage" {
        n175 = Unbundle By Name(w386) -> ("Queue Ref.Queue List"=w383:map{string, refnum<queue>}, "Queue Ref.Project Name"=w384:string)
        n176 = Concatenate Strings(w384, "-DMS" ("Name")) -> (w382:string)
        n177 = Look In Map(map=w383, key=w382) -> (value=w381:refnum<queue>)  [unwired: 1 in, 1 out]
        n178 = call "Queue In.vi"("Message"="Panel Show", "Queue In"=w381) -> ("error out"=w378:errorcluster, "Queue Out"=w379:refnum<queue>)  [unwired: 8 in]
        n179 = call "Queue In.vi"("error in (no error)"=w378, "Message"="Panel Max", "Queue In"=w379) -> ()  [unwired: 7 in, 2 out]
      }
      frame "FCTS DAQ" {
        n180 = call <vilib>:"System Exec.vi"("run minimized? (F)"=TRUE, "wait until completion? (T)"=FALSE, "command line"="CMD /C start http://127.0.0.1:9010/") -> ()  [unwired: 5 in, 4 out]
      }
      frame "Panel Name" {
        n181 = in-place {
          in-place-border: w402 -> [w408]
          n182 = in-place-cluster #7(w403) -> ("Panel Name"=w407:string[])
          n183 = Variant To Data(type=w407, Variant=w408) -> (data=w406:string[])  [unwired: 1 in, 1 out]
          n184 = in-place-cluster #7("Panel Name"=w406) -> (w401:T9)
        }
        n185 = Unbundle By Name(w401) -> ("Queue Ref.Queue List"=w399:map{string, refnum<queue>}, "Panel Adjust"=w398:string, "Panel Name"=w396:string[])
        n186 = Look In Map(map=w399, key=w398) -> (value=w397:refnum<queue>)  [unwired: 1 in, 1 out]
        n187 = call "Queue In.vi"("Data"=w396, "Message"=w400, "Queue In"=w397) -> ()  [unwired: 7 in, 2 out]
      }
      frame "Module Connect" {
        n188 = Unbundle By Name(w413) -> ("Panel Name"=w410:string[], "Panel Info"=w415:T10)
        n189 = for {
          tunnel: w410 -> [w422] mode=indexing
          tunnel: [w419] -> w409 mode=indexing
          n190 = call <vilib>:"Delimited String to 1D String Array.vi"("delimiter"="-", "delimited string"=w422) -> ("string array"=w420:string[])  [unwired: 9 in]
          n191 = Index Array(array=w420) -> (element #2=w419:string)  [unwired: 2 in, 1 out]
        }
        n192 = call "Module Connect.vi"("Panel Info In"=w415, "Panel Name"=w409) -> ("Panel Info Out"=w414:T10, "OK?"=w416:bool)  [unwired: 8 in]
        n193 = case shown="真" w416 {
          tunnel: w414 -> [_ w425]
          tunnel: w413 -> [w423 w427]
          tunnel: [w423 w426] -> w412
          tunnel: [_ "Panel Info Save,Panel Refresh" ("Message")] -> w411
          frame False {
          }
          frame True {
            n194 = Bundle By Name(cluster=w427, "Panel Info"=w425) -> (w426:T9)
          }
        }
      }
      frame "Panel Info Load" {
        n195 = Unbundle By Name(w438) -> ("Queue Ref.Data Path"=w431:path)
        n196 = Build Path(base path=w431, name or relative path=path "Config.csv" ("名称或相对路径")) -> (appended path=w430:path)
        n197 = call <vilib>:"Check if File or Folder Exists.vi"("path"=w430) -> ("file or folder exists?"=w428:bool, "dup path"=w429:path)  [unwired: 8 in, 1 out]
        n198 = case shown="真" w428 {
          tunnel: [_ w443] -> w437
          tunnel: w429 -> [_ w442]
          frame False {
          }
          frame True {
            n199 = call-poly <vilib>:"Read Delimited Spreadsheet.vi"("file path (dialog if empty)"=w442, "delimiter (\\t)"="," ("delimiter (\\t)")) -> ("all rows"=w443:string[][])  [unwired: 8 in, 5 out]
          }
        }
        n200 = Delete From Array(array=w437, length=1 ("长度"), index (row)=0 ("索引 (行)")) -> (array with subset deleted=w433:string[][])  [unwired: 1 in, 1 out]
        n201 = for {
          tunnel: w433 -> [w445] mode=indexing
          shift-right: [w446] -> w434
          shift-left: w438 -> [w447]
          n202 = in-place {
            in-place-border: w445 -> [w456]
            n203 = in-place-cluster #8(w447) -> ("Panel Info"=w450:T10)
            n204 = Index Array(array=w456) -> (element #1=w449:string, element #2=w455:string, element #3=w454:string, element #4=w453:string)  [unwired: 4 in]
            n205 = Look In Map(map=w450, key=w449) -> (value=w448:T11)  [unwired: 1 in, 1 out]
            n206 = Bundle By Name(cluster=w448, "Lable"=w449, "Name"=w455, "Panel"=w454, "Use"=w453) -> (w451:T11)
            n207 = Insert Into Map(map in=w450, key=w449, value=w451) -> (map out=w452:T10)  [unwired: 2 out]
            n208 = in-place-cluster #8("Panel Info"=w452) -> (w446:T9)
          }
        }
      }
      frame "Panel Info Save" {
        n209 = Unbundle By Name(w465) -> ("Panel Info"=w464:T10)
        n210 = for {
          tunnel: w464 -> [w471] mode=indexing
          tunnel: [w469] -> w463 mode=indexing
          n211 = Unbundle By Name(w471) -> ("Panel Info"=w470:T11)
          n212 = Cluster To Array(cluster=w470) -> (array=w469:string[])
        }
        n213 = Unbundle By Name(w465) -> ("Queue Ref.Data Path"=w457:path)
        n214 = Build Array (concatenate)(string[] ["Lable", "Text.Text", "Panel Name", "Enable"], w463) -> (w459:string[][])
        n215 = Build Path(base path=w457, name or relative path=path "Config.csv" ("名称或相对路径")) -> (appended path=w461:path)
        n216 = call-poly <vilib>:"Write Delimited Spreadsheet.vi"("file path (dialog if empty)"=w461, "2D data"=w459, "delimiter (\\t)"="," ("delimiter (\\t)")) -> ()  [unwired: 11 in, 2 out]
      }
      frame "Exit" {
        n217 = Unbundle By Name(w475) -> ("Queue Ref.UE"=w474:refnum<user-event>, "Queue Ref.Message"=w473:refnum<queue>, "Queue Ref.Data"=w472:refnum<queue>)
        n218 = Build Array(w473, w472) -> (w478:refnum<queue>[])
        n219 = for {
          tunnel: w478 -> [w485] mode=indexing
          tunnel: w477 -> [w484]
          n220 = call "Queue In.vi"("Message"=w484, "Queue In"=w485) -> ()  [unwired: 8 in, 2 out]
        }
        n221 = Generate User Event(user event=w474, event data cluster=w477) -> (error out=w476:errorcluster)  [unwired: 2 in, 1 out]
        n222 = call <vilib>:"Clear Errors.vi"("error in (no error)"=w476) -> ()  [unwired: 5 in, 2 out]
        n223 = call "Queue Clear.vi"("error in (no error)"=w480, "Queue In"=w482) -> ("error out"=w479:errorcluster, "Queue Out"=w481:refnum<queue>)  [unwired: 8 in]
      }
      frame "Quit" {
      }
    }
    n224 = call "Queue In.vi"("error in (no error)"=w314, "Data"=w312, "Message"=w313, "Queue In"=w317) -> ("error out"=w315:errorcluster, "Queue Out"=w316:refnum<queue>)  [unwired: 6 in]
  }
  n225 = call "000 Driver Message.vi"("Queue In"=w4) -> ("error out"=w22:errorcluster)  [unwired: 8 in, 2 out]
  n226 = call "Queue Release.vi"("error in (no error)"=w19, "Queue In"=w18) -> ("error out"=w21:errorcluster)  [unwired: 9 in]
  n227 = call "Queue Release.vi"("error in (no error)"=w11, "Queue In"=w10) -> ("error out"=w14:errorcluster)  [unwired: 9 in]
  n228 = Unregister For Events(event registration refnum=w8) -> (error out=w9:errorcluster)  [unwired: 1 in]
  n229 = Destroy User Event(user event=w6, error in=w9) -> (error out=w13:errorcluster)
  n230 = Call Chain() -> (call chain=w16:string[])
  n231 = Merge Errors(w13, w14, w22, w21) -> (w15:errorcluster)
  n232 = Array Size(array=w16) -> (size(s)=w17:i32)
  n233 = case shown="2.." w17 {
    tunnel: w15 -> [_ w490]
    frame 0, Default {
    }
    frame 2.. {
      n234 = invoke class="VI" method="FP.Close"(error in=w490) -> ()  [unwired: 2 in, 3 out]
    }
  }
